vi "Main.vi"() -> ()   [LabVIEW 2015]
doc: "使用该模板构建简单状态机设计模式。各状态执行代码并决定转移状态。"
uses:
  C:/Program Files (x86)/MVS/Development/DotNet/AnyCpu/MvCamCtrl.Net.dll
  DotNet/AnyCpu/MvCamCtrl.Net.dll
  controls/RetureState.ctl
panel:
  out "FrameNum":u32 caption="图像数"
  out "ResultingFrameRate":sgl caption="采集帧率："
  out "Processed Frame":dbl caption="处理帧率："
  out "?":T1(plugin-control)
  in  "SetParam":bool
  in  "GetParam":bool caption="获取参数"
  out "error out":T2 caption="错误输出" {"code" format="%x"}
  out "CFrameoutEx":refnum<k24>
  out "PayloadSize":u32 caption="帧负载大小："
  out "CFloatValue":refnum<k24>
  out "CEnumValue":refnum<k24>
  out "CIntValue":refnum<k24>
  out "Width":u32 caption="图像宽："
  out "Height":u32 caption="图像高："
  in  "error in":errorcluster caption="错误输入" {"code" format="%x"}
  out "CCameraInfoList":refnum<k24>
  in  "PixelFormat":u32 caption="像素格式" format="%x"
  in  "Gain":sgl caption="增益(dB)" min=0 max=20 format="%.4f"
  in  "ExposureTime":sgl=5.0 caption="曝光时间(us)" min=5 max=100000 format="%.4f"
  in  "TriggerSoftWare":bool
  in  "AcquisitionStop":bool
  in  "TriggerMode":bool
  in  "Continuous":bool
  in  "AcquisitionStart":bool caption="开始采集"
  out "GrabbingStatus":bool caption="图像采集"
  out "OpenSatatus":bool caption="相机打开"
  in  "退出":bool
  in  "CloseDevice":bool
  in  "OpenDevice":bool
  in  "EumDevice":bool
  in  "DeviceList":u16(ring) caption="设备列表" items=["[GigE]MV-CA013-20GC（Vir26769280）", "[GigE]MV-CA050-10GC（Vir26769488）", "[GigE]MV-CA060-11GM（Vir26769777）", "[GigE]MV-CL020-40GM（Vir26770200）", "[GigE]MV-CL042-91GC（Vir26770020）", "[U3V]MV-CA003-21UC（Vir26771277）", "[U3V]MV-CH120-10UC（Vir26771865）", "[U3V]MV-CH120-10UM（Vir26772137）"]
  out "DeviceNum":dbl caption="设备个数"
  out "CCamera":refnum<k24>
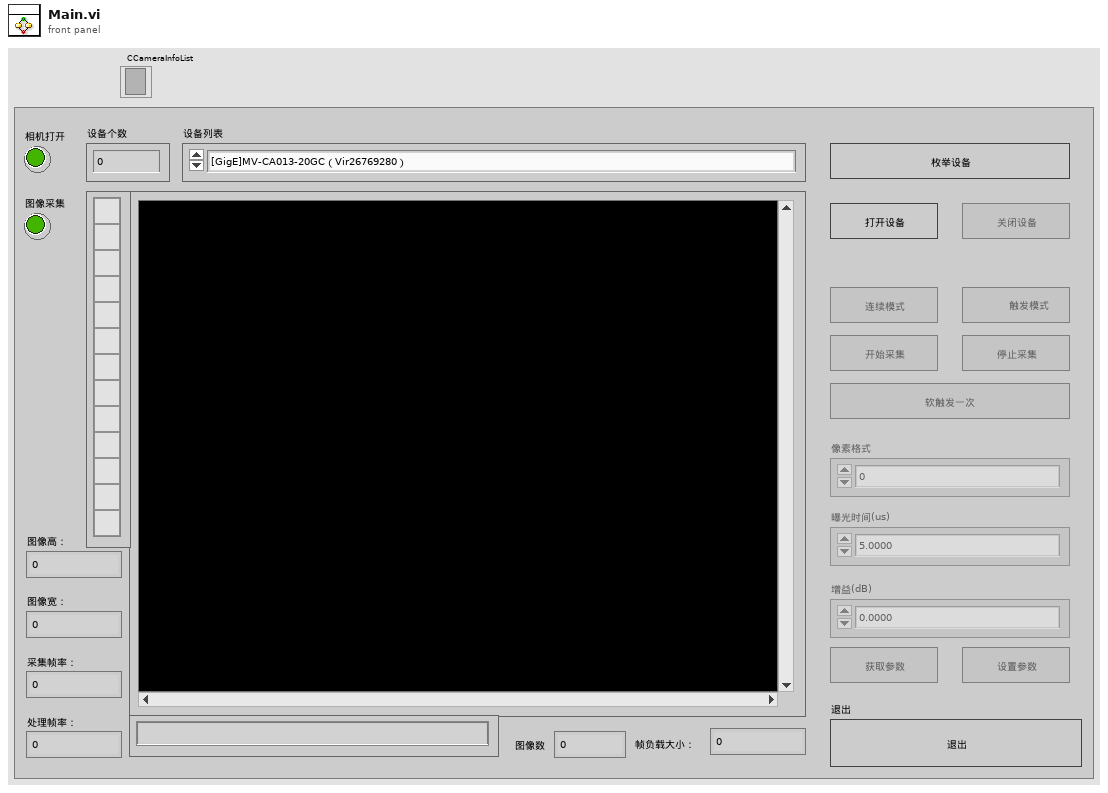
[diagram p1: front panel]
types:
  T1 = typedef "IMAQ Image.ctl" = refnum<image>
  T2 = typedef "RetureState.ctl" = errorcluster
  T3 = enum8{"Enabled", "Disabled", "Disabled and Grayed Out"}
  T4 = typedef "Image Type" = u32
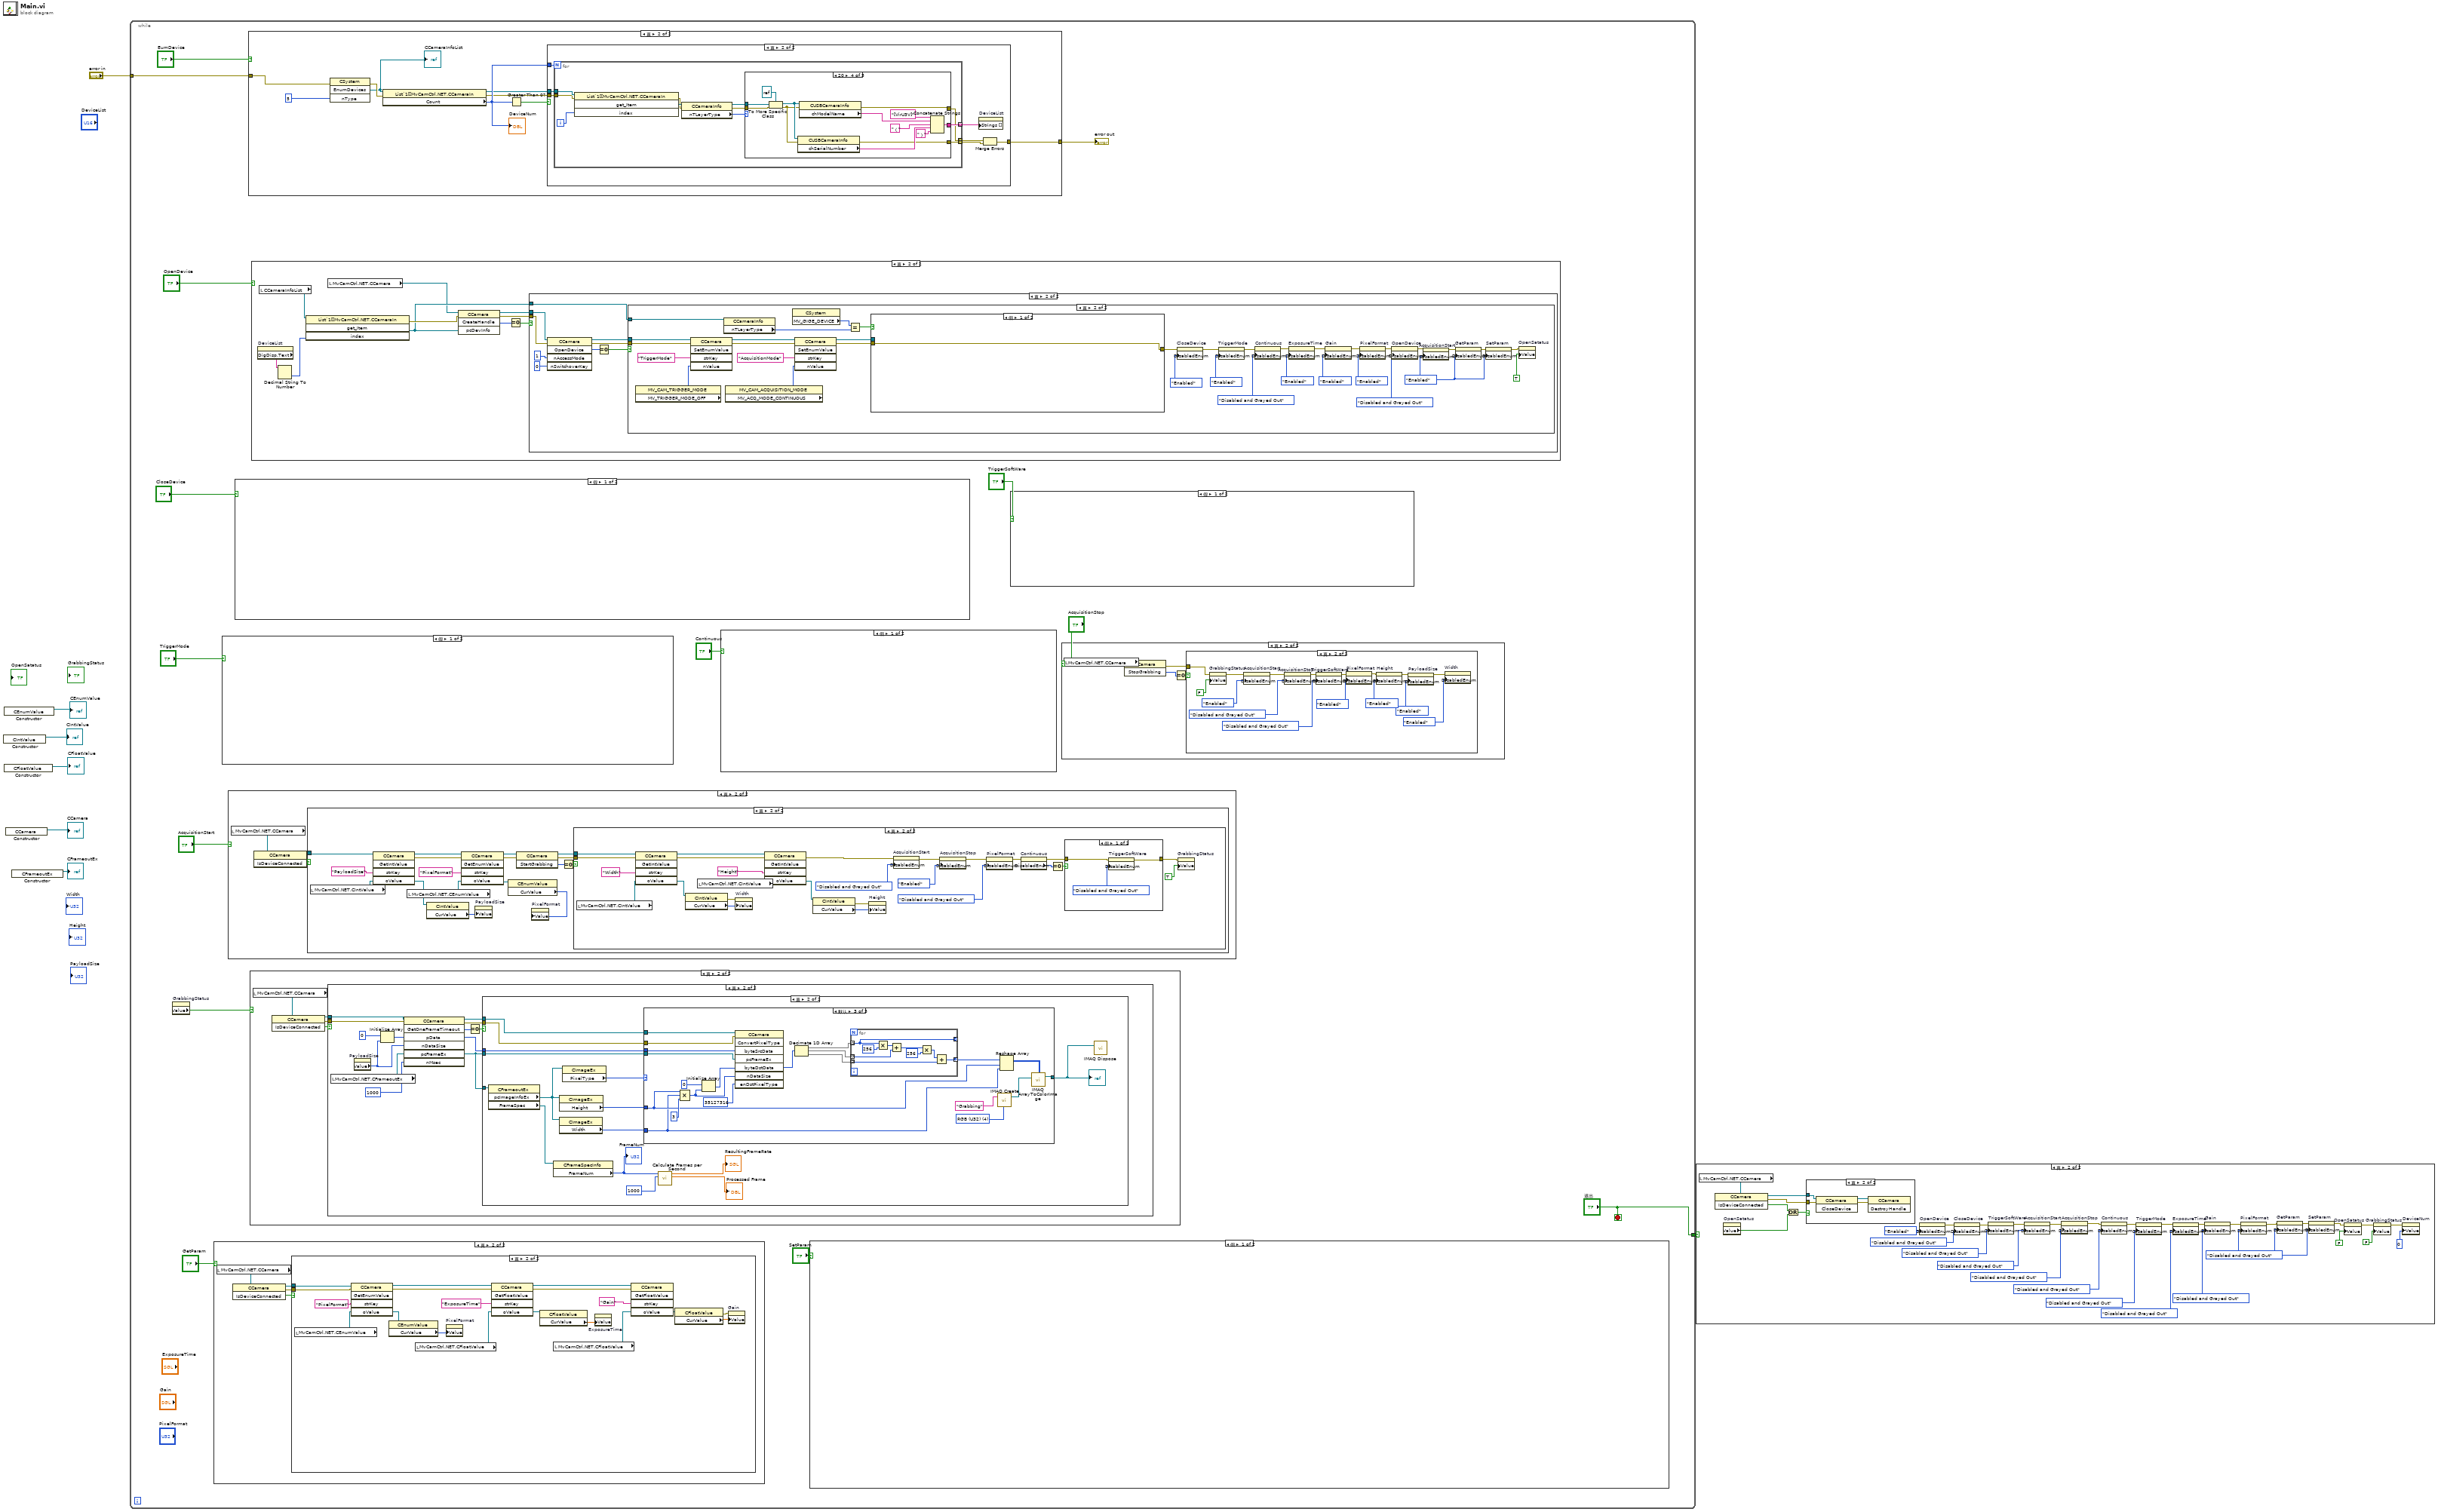
[diagram p0: block diagram]
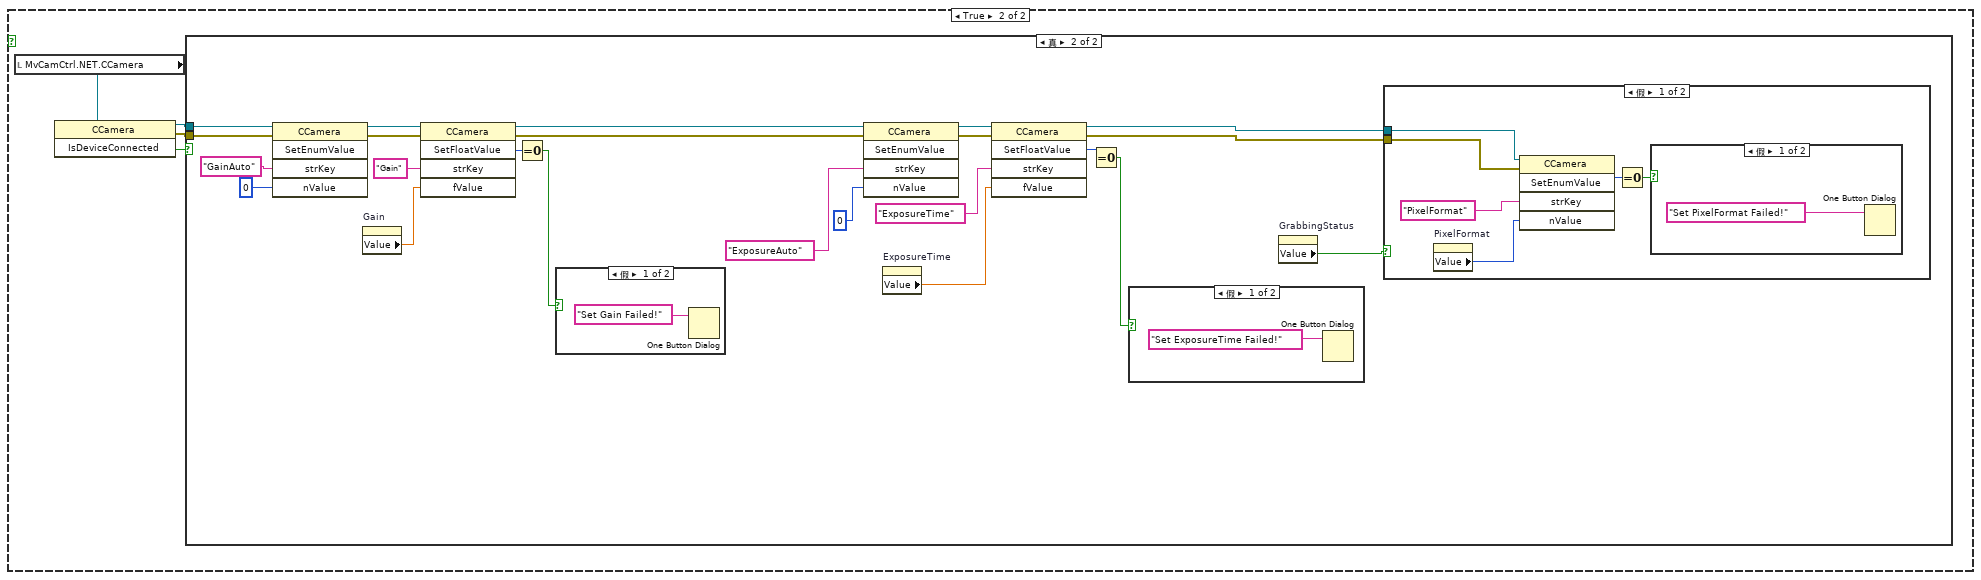
[diagram p4: hidden frame]
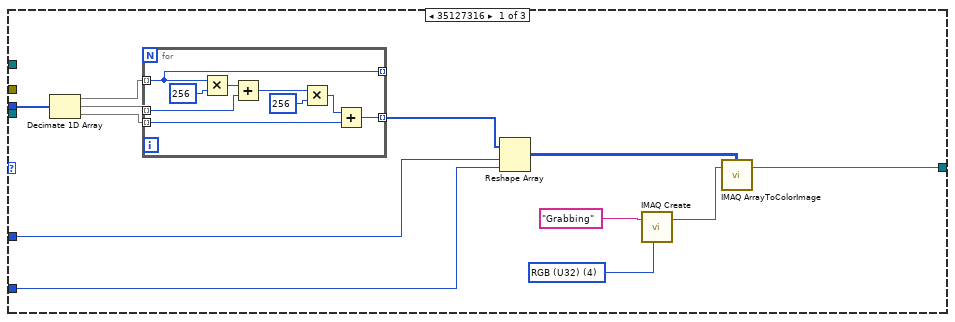
[diagram p15: hidden frame]
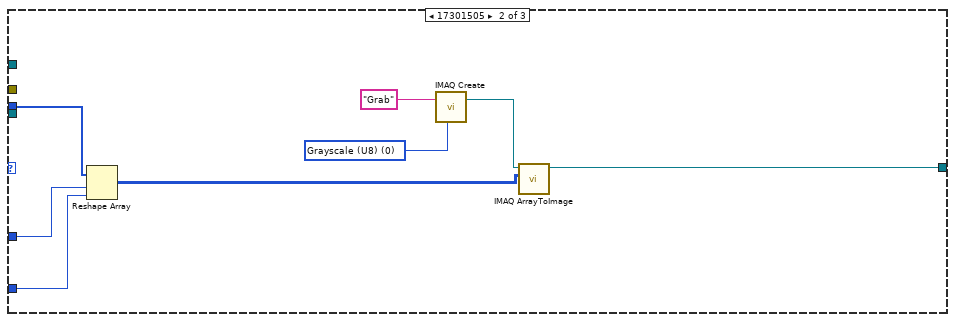
[diagram p16: hidden frame]
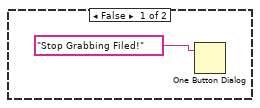
[diagram p18: hidden frame]
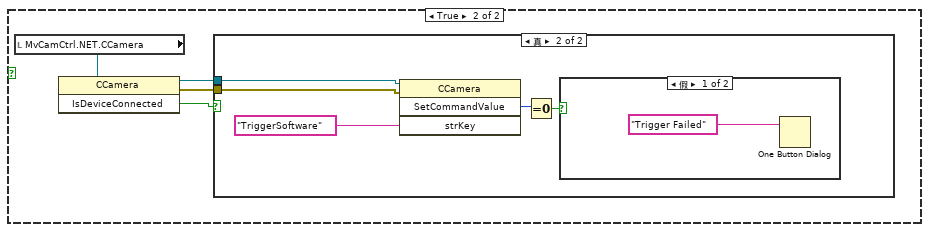
[diagram p19: hidden frame]
diagram:
  n1 = constructor class="CIntValue"() -> (reference out=→"CIntValue":refnum<k24>)  [unwired: 3 in, 2 out]
  n2 = constructor class="CEnumValue"() -> (reference out=→"CEnumValue":refnum<k24>)  [unwired: 3 in, 2 out]
  n3 = constructor class="CFloatValue"() -> (reference out=→"CFloatValue":refnum<k24>)  [unwired: 3 in, 2 out]
  n4 = constructor class="CCamera"() -> (reference out=→"CCamera":refnum<k24>)  [unwired: 3 in, 2 out]
  n5 = constructor class="CFrameoutEx"() -> (reference out=→"CFrameoutEx":refnum<k24>)  [unwired: 3 in, 2 out]
  n6 = while {
    tunnel: ["退出"] -> w7
    tunnel: "error in" -> [w13]
    stop <- "退出" stop-if-true
    n7 = property on="GrabbingStatus" class="Bool (严格)"() -> ("Value"=w12:bool)  [unwired: 2 in, 2 out]
    n8 = case shown="真" "GetParam" {
      frame False {
      }
      frame True {
        n9 = local read "CCamera"() -> (w61:refnum<k24>)
        n10 = invoke class="CCamera" method="IsDeviceConnected"(reference=w61) -> (reference out=w59:refnum<k24>, error out=w58:errorcluster, "IsDeviceConnected"=w60:bool)  [unwired: 2 in]
        n11 = case shown="真" w60 {
          tunnel: w59 -> [_ w71]
          tunnel: w58 -> [_ w70]
          frame False {
          }
          frame True {
            n12 = local read "CEnumValue"() -> (w72:refnum<k24>)
            n13 = invoke on="调用节点" class="CCamera" method="GetEnumValue"(reference=w71, error in=w70, "strKey"="PixelFormat", "oValue"=w72) -> (reference out=w78:refnum<k24>, error out=w75:errorcluster, "oValue"=w79:refnum<k24>)  [unwired: 1 in, 2 out]
            n14 = property on="属性节点" class="CEnumValue"(reference=w79) -> ("CurValue"=w80:u32)  [unwired: 1 in, 2 out]
            n15 = local read "CFloatValue"() -> (w69:refnum<k24>)
            n16 = property on="PixelFormat" class="DigNum (严格)"("Value"=w80) -> ()  [unwired: 2 in, 2 out]
            n17 = invoke on="调用节点" class="CCamera" method="GetFloatValue"(reference=w78, error in=w75, "strKey"="ExposureTime", "oValue"=w69) -> (reference out=w77:refnum<k24>, error out=w74:errorcluster, "oValue"=w63:refnum<k24>)  [unwired: 1 in, 2 out]
            n18 = property on="属性节点" class="CFloatValue"(reference=w63) -> ("CurValue"=w62:sgl)  [unwired: 1 in, 2 out]
            n19 = local read "CFloatValue"() -> (w66:refnum<k24>)
            n20 = property on="ExposureTime" class="DigNum (严格)"("Value"=w62) -> ()  [unwired: 2 in, 2 out]
            n21 = invoke on="调用节点" class="CCamera" method="GetFloatValue"(reference=w77, error in=w74, "strKey"="Gain", "oValue"=w66) -> ("oValue"=w76:refnum<k24>)  [unwired: 1 in, 4 out]
            n22 = property on="属性节点" class="CFloatValue"(reference=w76) -> (error out=w65:errorcluster, "CurValue"=w64:sgl)  [unwired: 1 in, 1 out]
            n23 = property on="Gain" class="DigNum (严格)"(error in=w65, "Value"=w64) -> ()  [unwired: 1 in, 2 out]
          }
        }
      }
    }
    n24 = case shown="假" "TriggerMode" {
      frame False {
      }
      frame True {
        n25 = local read "CCamera"() -> (w222:refnum<k24>)
        n26 = property class="MV_CAM_TRIGGER_MODE"() -> ("MV_TRIGGER_MODE_ON"=w221:i32)  [unwired: 2 in, 2 out]
        n27 = invoke class="CCamera" method="SetEnumValue"(reference=w222, "strKey"="TriggerMode", "nValue"=w221) -> (reference out=w220:refnum<k24>, error out=w219:errorcluster, "SetEnumValue"=w217:i32)  [unwired: 2 in, 2 out]
        n28 = Equal To 0?(x=w217) -> (x = 0?=w218:bool)
        n29 = case shown="真" w218 {
          tunnel: w220 -> [_ w233]
          tunnel: w219 -> [_ w232]
          frame False {
            n30 = One Button Dialog(message="Set TiggerMode Filed!") -> ()  [unwired: 1 in, 1 out]
          }
          frame True {
            n31 = property class="MV_CAM_TRIGGER_SOURCE"() -> ("MV_TRIGGER_SOURCE_SOFTWARE"=w225:i32)  [unwired: 2 in, 2 out]
            n32 = invoke class="CCamera" method="SetEnumValue"(reference=w233, error in=w232, "strKey"="TriggerSource", "nValue"=w225) -> (error out=w231:errorcluster)  [unwired: 1 in, 4 out]
            n33 = property on="Continuous" class="Bool"(error in=w231, "DisabledEnum"=T3."Enabled" ("禁用")) -> (error out=w230:errorcluster)  [unwired: 1 in, 1 out]
            n34 = property on="TriggerMode" class="Bool"(error in=w230, "DisabledEnum"=T3."Disabled and Grayed Out" ("禁用")) -> (error out=w229:errorcluster)  [unwired: 1 in, 1 out]
            n35 = property on="TriggerSoftWare" class="Bool"(error in=w229, "DisabledEnum"=T3."Enabled" ("禁用")) -> ()  [unwired: 1 in, 2 out]
          }
        }
      }
    }
    n36 = case shown="真" "AcquisitionStart" {
      frame False {
      }
      frame True {
        n37 = local read "CCamera"() -> (w236:refnum<k24>)
        n38 = invoke class="CCamera" method="IsDeviceConnected"(reference=w236) -> (reference out=w234:refnum<k24>, "IsDeviceConnected"=w235:bool)  [unwired: 2 in, 1 out]
        n39 = case shown="真" w235 {
          tunnel: w234 -> [_ w238]
          frame False {
          }
          frame True {
            n40 = local read "CIntValue"() -> (w249:refnum<k24>)
            n41 = invoke class="CCamera" method="GetIntValue"(reference=w238, "strKey"="PayloadSize", "oValue"=w249) -> (reference out=w244:refnum<k24>, error out=w242:errorcluster, "oValue"=w253:refnum<k24>)  [unwired: 2 in, 2 out]
            n42 = local read "CEnumValue"() -> (w247:refnum<k24>)
            n43 = property class="CIntValue"(reference=w253) -> ("CurValue"=w248:i64)  [unwired: 1 in, 2 out]
            n44 = invoke on="调用节点" class="CCamera" method="GetEnumValue"(reference=w244, error in=w242, "strKey"="PixelFormat", "oValue"=w247) -> (reference out=w243:refnum<k24>, error out=w241:errorcluster, "oValue"=w246:refnum<k24>)  [unwired: 1 in, 2 out]
            n45 = property on="PayloadSize" class="DigNum (严格)"("Value"=w248) -> ()  [unwired: 2 in, 2 out]
            n46 = property class="CEnumValue"(reference=w246) -> ("CurValue"=w245:u32)  [unwired: 1 in, 2 out]
            n47 = invoke class="CCamera" method="StartGrabbing"(reference=w243, error in=w241) -> (reference out=w251:refnum<k24>, error out=w250:errorcluster, "StartGrabbing"=w237:i32)  [unwired: 1 in]
            n48 = property on="PixelFormat" class="DigNum (严格)"("Value"=w245) -> ()  [unwired: 2 in, 2 out]
            n49 = Equal To 0?(x=w237) -> (x = 0?=w252:bool)
            n50 = case shown="真" w252 {
              tunnel: w251 -> [_ w280]
              tunnel: w250 -> [_ w277]
              frame False {
                n51 = One Button Dialog(message="Satrt Grabbing Failed") -> ()  [unwired: 1 in, 1 out]
              }
              frame True {
                n52 = local read "CIntValue"() -> (w258:refnum<k24>)
                n53 = invoke class="CCamera" method="GetIntValue"(reference=w280, error in=w277, "strKey"="Width", "oValue"=w258) -> (reference out=w279:refnum<k24>, error out=w278:errorcluster, "oValue"=w275:refnum<k24>)  [unwired: 1 in, 2 out]
                n54 = property class="CIntValue"(reference=w275) -> (error out=w276:errorcluster, "CurValue"=w274:i64)  [unwired: 1 in, 1 out]
                n55 = local read "CIntValue"() -> (w257:refnum<k24>)
                n56 = property on="Width" class="DigNum (严格)"(error in=w276, "Value"=w274) -> ()  [unwired: 1 in, 2 out]
                n57 = invoke class="CCamera" method="GetIntValue"(reference=w279, error in=w278, "strKey"="Height", "oValue"=w257) -> (error out=w260:errorcluster, "oValue"=w264:refnum<k24>)  [unwired: 1 in, 3 out]
                n58 = property class="CIntValue"(reference=w264) -> (error out=w273:errorcluster, "CurValue"=w272:i64)  [unwired: 1 in, 1 out]
                n59 = property on="Height" class="DigNum (严格)"(error in=w273, "Value"=w272) -> ()  [unwired: 1 in, 2 out]
                n60 = property on="AcquisitionStart" class="Bool"(error in=w260, "DisabledEnum"=T3."Disabled and Grayed Out" ("禁用")) -> (error out=w271:errorcluster)  [unwired: 1 in, 1 out]
                n61 = property on="AcquisitionStop" class="Bool"(error in=w271, "DisabledEnum"=T3."Enabled" ("禁用")) -> (error out=w263:errorcluster)  [unwired: 1 in, 1 out]
                n62 = property on="PixelFormat" class="DigNum (严格)"(error in=w263, "DisabledEnum"=T3."Disabled and Grayed Out" ("禁用")) -> (error out=w259:errorcluster)  [unwired: 1 in, 1 out]
                n63 = property on="Continuous" class="Bool"(error in=w259) -> (error out=w270:errorcluster, "DisabledEnum"=w265:T3)  [unwired: 1 in, 1 out]
                n64 = Equal To 0?(x=w265) -> (x = 0?=w266:bool)
                n65 = case shown="假" w266 {
                  tunnel: w270 -> [w282 w286]
                  tunnel: [w281 w285] -> w268
                  frame False {
                    n66 = property on="TriggerSoftWare" class="Bool"(error in=w282, "DisabledEnum"=T3."Disabled and Grayed Out" ("禁用")) -> (error out=w281:errorcluster)  [unwired: 1 in, 1 out]
                  }
                  frame True {
                    n67 = property on="TriggerSoftWare" class="Bool"(error in=w286, "DisabledEnum"=T3."Enabled" ("禁用")) -> (error out=w285:errorcluster)  [unwired: 1 in, 1 out]
                  }
                }
                n68 = property on="GrabbingStatus" class="Bool (严格)"(error in=w268, "Value"=TRUE) -> ()  [unwired: 1 in, 2 out]
              }
            }
          }
        }
      }
    }
    n69 = case shown="假" "CloseDevice" {
      frame False {
      }
      frame True {
        n70 = local read "CCamera"() -> (w448:refnum<k24>)
        n71 = invoke class="CCamera" method="IsDeviceConnected"(reference=w448) -> (reference out=w447:refnum<k24>, error out=w446:errorcluster, "IsDeviceConnected"=w445:bool)  [unwired: 2 in]
        n72 = case shown="真" w445 {
          tunnel: w447 -> [_ w454]
          tunnel: w446 -> [_ w453]
          frame False {
          }
          frame True {
            w452 = T3."Disabled and Grayed Out" ("禁用")
            n73 = invoke class="CCamera" method="CloseDevice"(reference=w454, error in=w453) -> (reference out=w478:refnum<k24>, error out=w477:errorcluster)  [unwired: 1 in, 1 out]
            n74 = invoke class="CCamera" method="DestroyHandle"(reference=w478, error in=w477) -> (error out=w476:errorcluster)  [unwired: 1 in, 2 out]
            n75 = property on="OpenDevice" class="Bool"(error in=w476, "DisabledEnum"=T3."Enabled" ("禁用")) -> (error out=w472:errorcluster)  [unwired: 1 in, 1 out]
            n76 = property on="CloseDevice" class="Bool"(error in=w472, "DisabledEnum"=T3."Disabled and Grayed Out" ("禁用")) -> (error out=w471:errorcluster)  [unwired: 1 in, 1 out]
            n77 = property on="Continuous" class="Bool"(error in=w471, "DisabledEnum"=T3."Disabled and Grayed Out" ("禁用")) -> (error out=w470:errorcluster)  [unwired: 1 in, 1 out]
            n78 = property on="TriggerMode" class="Bool"(error in=w470, "DisabledEnum"=T3."Disabled and Grayed Out" ("禁用")) -> (error out=w457:errorcluster)  [unwired: 1 in, 1 out]
            n79 = property on="AcquisitionStop" class="Bool"(error in=w457, "DisabledEnum"=T3."Disabled and Grayed Out" ("禁用")) -> (error out=w469:errorcluster)  [unwired: 1 in, 1 out]
            n80 = property on="AcquisitionStart" class="Bool"(error in=w469, "DisabledEnum"=T3."Disabled and Grayed Out" ("禁用")) -> (error out=w455:errorcluster)  [unwired: 1 in, 1 out]
            n81 = property on="TriggerSoftWare" class="Bool"(error in=w455, "DisabledEnum"=T3."Disabled and Grayed Out" ("禁用")) -> (error out=w459:errorcluster)  [unwired: 1 in, 1 out]
            n82 = property on="PixelFormat" class="DigNum (严格)"(error in=w459, "DisabledEnum"=T3."Disabled and Grayed Out" ("禁用")) -> (error out=w458:errorcluster)  [unwired: 1 in, 1 out]
            n83 = property on="Gain" class="DigNum (严格)"(error in=w458, "DisabledEnum"=T3."Disabled and Grayed Out" ("禁用")) -> (error out=w468:errorcluster)  [unwired: 1 in, 1 out]
            n84 = property on="ExposureTime" class="DigNum (严格)"(error in=w468, "DisabledEnum"=w452) -> (error out=w451:errorcluster)  [unwired: 1 in, 1 out]
            n85 = property on="GetParam" class="Bool"(error in=w451, "DisabledEnum"=w452) -> (error out=w450:errorcluster)  [unwired: 1 in, 1 out]
            n86 = property on="SetParam" class="Bool"(error in=w450, "DisabledEnum"=w452) -> (error out=w449:errorcluster)  [unwired: 1 in, 1 out]
            n87 = property on="OpenSatatus" class="Bool (严格)"(error in=w449, "Value"=FALSE) -> (error out=w460:errorcluster)  [unwired: 1 in, 1 out]
            n88 = property on="GrabbingStatus" class="Bool (严格)"(error in=w460, "Value"=FALSE) -> ()  [unwired: 1 in, 2 out]
          }
        }
      }
    }
    n89 = case shown="真" "EumDevice" {
      tunnel: w13 -> [w360 w367]
      tunnel: [w360 w364] -> w11
      frame False {
      }
      frame True {
        n90 = invoke on="调用节点" class="CSystem" method="EnumDevices"(error in=w367, "nType"=u32 5) -> (error out=w366:errorcluster, "EnumDevices"=w361:refnum<k24>)  [unwired: 2 in, 2 out]
        "CCameraInfoList" <- w361
        n91 = property on="属性节点" class="List`1[[MvCamCtrl.NET.CCameraIn"(reference=w361, error in=w366) -> (reference out=w363:refnum<k24>, error out=w365:errorcluster, "Count"=w368:i32)
        "DeviceNum" <- w368
        n92 = Greater Than 0?(x=w368) -> (x > 0?=w369:bool)
        n93 = case shown="真" w369 {
          tunnel: w368 -> [_ w379]
          tunnel: w363 -> [_ w378]
          tunnel: w365 -> [w370 w376]
          tunnel: [w370 w373] -> w364
          frame False {
            n94 = One Button Dialog(message="Not Found Devices!", button name ("OK")="Warning") -> ()  [unwired: 1 out]
          }
          frame True {
            n95 = for {
              N: w379 -> [_]
              tunnel: [w390] -> w377 mode=indexing
              tunnel: w378 -> [w385]
              tunnel: w376 -> [w384]
              tunnel: [w381] -> w375 mode=indexing
              tunnel: [w380] -> w374 mode=indexing
              i -> [w389]
              n96 = invoke class="List`1[[MvCamCtrl.NET.CCameraIn" method="get_Item"(reference=w385, error in=w384, "index"=w389) -> (error out=w383:errorcluster, "get_Item"=w386:refnum<k24>)  [unwired: 1 in, 2 out]
              n97 = property class="CCameraInfo"(reference=w386, error in=w383) -> (reference out=w387:refnum<k24>, error out=w382:errorcluster, "nTLayerType"=w388:u32)
              n98 = case shown="20" w388 {
                tunnel: ["UnsupportDev" w402 w406 w419 w439] -> w390
                tunnel: w387 -> [_ w398 w410 w423 w437]
                tunnel: w382 -> [w391 w396 w409 w422 w433]
                tunnel: [w391 w394 w407 w421 w435] -> w381
                tunnel: [w391 w393 w408 w420 w434] -> w380
                frame 0, Default {
                }
                frame 1 {
                  n99 = To More Specific Class(target class=refnum<k24> refnum ("CGigECameraInfo"), reference=w398, error in=w396) -> (specific class reference=w397:refnum<k24>, error out=w395:errorcluster)
                  n100 = property class="CGigECameraInfo"(reference=w397, error in=w395) -> (error out=w394:errorcluster, "chModelName"=w401:string)  [unwired: 1 out]
                  n101 = property class="CGigECameraInfo"(reference=w397, error in=w395) -> (error out=w393:errorcluster, "chSerialNumber"=w403:string)  [unwired: 1 out]
                  n102 = Concatenate Strings("[GigE]" ("字符串"), w401, "（" ("字符串"), w403, "）" ("字符串")) -> (w402:string)
                }
                frame 16 {
                  n103 = To More Specific Class(target class=refnum<k24> refnum ("CGigECameraInfo"), reference=w410, error in=w409) -> (specific class reference=w412:refnum<k24>, error out=w411:errorcluster)
                  n104 = property class="CGigECameraInfo"(reference=w412, error in=w411) -> (error out=w407:errorcluster, "chModelName"=w415:string)  [unwired: 1 out]
                  n105 = property class="CGigECameraInfo"(reference=w412, error in=w411) -> (error out=w408:errorcluster, "chSerialNumber"=w416:string)  [unwired: 1 out]
                  n106 = Concatenate Strings("[VirGigE]" ("字符串"), w415, "（" ("字符串"), w416, "）" ("字符串")) -> (w406:string)
                }
                frame 32 {
                  n107 = To More Specific Class(target class=refnum<k24> refnum ("CUSBCameraInfo"), reference=w423, error in=w422) -> (specific class reference=w425:refnum<k24>, error out=w424:errorcluster)
                  n108 = property class="CUSBCameraInfo"(reference=w425, error in=w424) -> (error out=w420:errorcluster, "chSerialNumber"=w429:string)  [unwired: 1 out]
                  n109 = property class="CUSBCameraInfo"(reference=w425, error in=w424) -> (error out=w421:errorcluster, "chModelName"=w428:string)  [unwired: 1 out]
                  n110 = Concatenate Strings("[VirU3V]" ("字符串"), w428, "（" ("字符串"), w429, "）" ("字符串")) -> (w419:string)
                }
                frame 4 {
                  n111 = To More Specific Class(target class=refnum<k24> refnum ("CUSBCameraInfo"), reference=w437, error in=w433) -> (specific class reference=w436:refnum<k24>, error out=w432:errorcluster)
                  n112 = property class="CUSBCameraInfo"(reference=w436, error in=w432) -> (error out=w434:errorcluster, "chSerialNumber"=w442:string)  [unwired: 1 out]
                  n113 = property class="CUSBCameraInfo"(reference=w436, error in=w432) -> (error out=w435:errorcluster, "chModelName"=w441:string)  [unwired: 1 out]
                  n114 = Concatenate Strings("[U3V]" ("字符串"), w441, "（" ("字符串"), w442, "）" ("字符串")) -> (w439:string)
                }
              }
            }
            n115 = property on="DeviceList" class="Ring (严格)"("Strings []"=w377) -> ()  [unwired: 2 in, 2 out]
            n116 = Merge Errors(w375, w374) -> (w373:errorcluster)
          }
        }
      }
    }
    "error out" <- w11
    n117 = case shown="真" w12 {
      frame False {
      }
      frame True {
        n118 = local read "CCamera"() -> (w84:refnum<k24>)
        n119 = invoke class="CCamera" method="IsDeviceConnected"(reference=w84) -> (reference out=w82:refnum<k24>, error out=w81:errorcluster, "IsDeviceConnected"=w83:bool)  [unwired: 2 in]
        n120 = case shown="真" w83 {
          tunnel: w82 -> [_ w89]
          tunnel: w81 -> [_ w88]
          frame False {
          }
          frame True {
            n121 = local read "CFrameoutEx"() -> (w95:refnum<k24>)
            n122 = property on="PayloadSize" class="DigNum (严格)"() -> ("Value"=w91:u32)  [unwired: 2 in, 2 out]
            n123 = Initialize Array(0, w91) -> (w93:i32[])
            n124 = invoke class="CCamera" method="GetOneFrameTimeout"(reference=w89, error in=w88, "pData"=w93, "nDataSize"=w91, "pcFrameEx"=w95, "nMsec"=1000) -> (reference out=w87:refnum<k24>, error out=w94:errorcluster, "GetOneFrameTimeout"=w97:i32, "pData"=w90:u8[], "pcFrameEx"=w86:refnum<k24>)  [unwired: 1 in, 2 out]
            n125 = Equal To 0?(x=w97) -> (x = 0?=w96:bool)
            n126 = case shown="真" w96 {
              tunnel: w86 -> [_ w111]
              tunnel: w94 -> [_ w112]
              tunnel: w90 -> [_ w105]
              tunnel: w87 -> [_ w103]
              tunnel: w86 -> [_ w102]
              frame False {
              }
              frame True {
                n127 = property on="属性节点" class="CFrameoutEx"(reference=w111) -> ("pcImageInfoEx"=w107:refnum<k24>, "FrameSpec"=w104:refnum<k24>)  [unwired: 1 in, 2 out]
                n128 = property on="属性节点" class="CFrameSpecInfo"(reference=w104) -> ("FrameNum"=w101:u32)  [unwired: 1 in, 2 out]
                "FrameNum" <- w101
                n129 = property on="属性节点" class="CImageEx"(reference=w107) -> ("Width"=w110:u16)  [unwired: 1 in, 2 out]
                n130 = property on="属性节点" class="CImageEx"(reference=w107) -> ("Height"=w109:u16)  [unwired: 1 in, 2 out]
                n131 = property on="属性节点" class="CImageEx"(reference=w107) -> ("PixelType"=w108:i32)  [unwired: 1 in, 2 out]
                n132 = case shown="默认" w108 {
                  tunnel: w105 -> [w120 w141 w155]
                  tunnel: w109 -> [w115 w140 w143]
                  tunnel: w110 -> [w114 w139 w142]
                  tunnel: w112 -> [_ _ w152]
                  tunnel: [w124 w134 w161] -> w106
                  tunnel: w103 -> [_ _ w156]
                  tunnel: w102 -> [_ _ w145]
                  frame 35127316 {
                    w122 = T4 4 items=["Grayscale (U8)", "Grayscale (I16)", "Grayscale (SGL)", "Complex (CSG)", "RGB (U32)", "HSL (U32)", "RGB (U64)", "Grayscale (U16)"] ("Image Type")
                    n133 = Decimate 1D Array(w120) -> (w119:u8[], w118:u8[], w117:u8[])
                    n134 = for {
                      tunnel: [w125] -> _ mode=indexing
                      tunnel: w118 -> [w128] mode=indexing
                      tunnel: w117 -> [w127] mode=indexing
                      tunnel: [w126] -> w116 mode=indexing
                      tunnel: w119 -> [w125] mode=indexing
                      n135 = Multiply(x=w125, y=u16 256) -> (x*y=w132:u16)
                      n136 = Add(x=w132, y=w128) -> (x+y=w129:u16)
                      n137 = Multiply ("乘")(x=w129, y=u16 256) -> (x*y=w131:u32)
                      n138 = Add(x=w131, y=w127) -> (x+y=w126:u32)
                    }
                    n139 = Reshape Array(w116, w115, w114) -> (w113:u32[][])
                    n140 = call "IMAQ Create"("Image Name"="Grabbing", "Image Type"=w122) -> ("New Image"=w121:T1)  [unwired: 3 in, 1 out]
                    n141 = call "IMAQ ArrayToColorImage"("Image Pixels (U32)"=w113, "Image"=w121) -> ("Image Out"=w124:T1)  [unwired: 3 in, 1 out]
                  }
                  frame 17301505 {
                    w137 = T4 0 items=["Grayscale (U8)", "Grayscale (I16)", "Grayscale (SGL)", "Complex (CSG)", "RGB (U32)", "HSL (U32)", "RGB (U64)", "Grayscale (U16)"] ("Image Type")
                    n142 = Reshape Array(w141, w140, w139) -> (w135:u8[][])
                    n143 = call "IMAQ Create"("Image Name"="Grab", "Image Type"=w137) -> ("New Image"=w136:T1)  [unwired: 3 in, 1 out]
                    n144 = call "IMAQ ArrayToImage"("Image Pixels (U8)"=w135, "Image"=w136) -> ("Image Out"=w134:T1)  [unwired: 8 in, 1 out]
                  }
                  frame Default {
                    w159 = T4 4 items=["Grayscale (U8)", "Grayscale (I16)", "Grayscale (SGL)", "Complex (CSG)", "RGB (U32)", "HSL (U32)", "RGB (U64)", "Grayscale (U16)"] ("Image Type")
                    n145 = Compound Arithmetic op=MULTIPLY(w143, w142, 3) -> (w153:i32)
                    n146 = Initialize Array(0, w153) -> (w154:i32[])
                    n147 = invoke class="CCamera" method="ConvertPixelType"(reference=w156, error in=w152, "byteSrcData"=w155, "pcFrameEx"=w145, "byteDstData"=w154, "nDataSize"=w153, "enDstPixelType"=u32 35127316) -> ("byteDstData"=w144:u8[])  [unwired: 1 in, 7 out]
                    n148 = Decimate 1D Array(w144) -> (w149:u8[], w148:u8[], w147:u8[])
                    n149 = for {
                      tunnel: [w163] -> _ mode=indexing
                      tunnel: w148 -> [w166] mode=indexing
                      tunnel: w147 -> [w165] mode=indexing
                      tunnel: [w164] -> w157 mode=indexing
                      tunnel: w149 -> [w163] mode=indexing
                      n150 = Multiply(x=w163, y=u16 256) -> (x*y=w170:u16)
                      n151 = Add(x=w170, y=w166) -> (x+y=w167:u16)
                      n152 = Multiply ("乘")(x=w167, y=u16 256) -> (x*y=w169:u32)
                      n153 = Add(x=w169, y=w165) -> (x+y=w164:u32)
                    }
                    n154 = call "IMAQ Create"("Image Name"="Grabbing", "Image Type"=w159) -> ("New Image"=w162:T1)  [unwired: 3 in, 1 out]
                    n155 = Reshape Array(w157, w143, w142) -> (w158:u32[][])
                    n156 = call "IMAQ ArrayToColorImage"("Image Pixels (U32)"=w158, "Image"=w162) -> ("Image Out"=w161:T1)  [unwired: 3 in, 1 out]
                  }
                }
                "?" <- w106
                n157 = call <vilib>:"Calculate Frames per Second.vi"("Update Interval (ms)"=1000, "Buffer Number"=w101) -> ("Processed Frames/s"=→"Processed Frame":dbl, "Acquired Frames/s"=→"ResultingFrameRate":dbl)  [unwired: 7 in, 1 out]
                n158 = call "IMAQ Dispose"("Image"=w106) -> ()  [unwired: 5 in, 1 out]
              }
            }
          }
        }
      }
    }
    n159 = case shown="真" "OpenDevice" {
      frame False {
      }
      frame True {
        n160 = property on="DeviceList" class="Ring (严格)"() -> ("DigDisp.Text"=w296:string)  [unwired: 2 in, 2 out]
        n161 = local read "CCameraInfoList"() -> (w287:refnum<k24>)
        n162 = Decimal String To Number(string=w296) -> (number=w295:i32)  [unwired: 2 in, 1 out]
        n163 = invoke class="List`1[[MvCamCtrl.NET.CCameraIn" method="get_Item"(reference=w287, "index"=w295) -> (error out=w294:errorcluster, "get_Item"=w293:refnum<k24>)  [unwired: 2 in, 2 out]
        n164 = local read "CCamera"() -> (w291:refnum<k24>)
        n165 = invoke class="CCamera" method="CreateHandle"(reference=w291, error in=w294, "pcDevInfo"=w293) -> (reference out=w292:refnum<k24>, error out=w290:errorcluster, "CreateHandle"=w289:i32)  [unwired: 1 in, 1 out]
        n166 = Equal To 0?(x=w289) -> (x = 0?=w288:bool)
        n167 = case shown="真" w288 {
          tunnel: w290 -> [_ w301]
          tunnel: w293 -> [_ w300]
          tunnel: w292 -> [_ w299]
          frame False {
            n168 = One Button Dialog(message="Create Camera Handle Failed!") -> ()  [unwired: 1 in, 1 out]
          }
          frame True {
            n169 = invoke class="CCamera" method="OpenDevice"(reference=w299, error in=w301, "nAccessMode"=1, "nSwitchoverKey"=0) -> (reference out=w303:refnum<k24>, error out=w302:errorcluster, "OpenDevice"=w298:i32)  [unwired: 1 in, 2 out]
            n170 = Equal To 0?(x=w298) -> (x = 0?=w306:bool)
            n171 = case shown="真" w306 {
              tunnel: w303 -> [w311 w345]
              tunnel: w302 -> [w310 w344]
              tunnel: w300 -> [_ w321]
              frame False {
                n172 = invoke class="CCamera" method="DestroyHandle"(reference=w311, error in=w310) -> (error out=w307:errorcluster)  [unwired: 1 in, 2 out]
                n173 = One Button Dialog(message="Open Failed") -> ()  [unwired: 1 in, 1 out]
                n174 = property on="OpenSatatus" class="Bool (严格)"(error in=w307, "Value"=FALSE) -> ()  [unwired: 1 in, 2 out]
              }
              frame True {
                w312 = T3."Enabled" ("禁用")
                n175 = property class="MV_CAM_TRIGGER_MODE"() -> ("MV_TRIGGER_MODE_OFF"=w338:i32)  [unwired: 2 in, 2 out]
                n176 = invoke class="CCamera" method="SetEnumValue"(reference=w345, error in=w344, "strKey"="TriggerMode", "nValue"=w338) -> (reference out=w340:refnum<k24>, error out=w339:errorcluster)  [unwired: 1 in, 3 out]
                n177 = property on="属性节点" class="CCameraInfo"(reference=w321) -> ("nTLayerType"=w343:u32)  [unwired: 1 in, 2 out]
                n178 = property class="MV_CAM_ACQUISITION_MODE"() -> ("MV_ACQ_MODE_CONTINUOUS"=w336:i32)  [unwired: 2 in, 2 out]
                n179 = property class="CSystem"() -> ("MV_GIGE_DEVICE"=w335:i32)  [unwired: 2 in, 2 out]
                n180 = invoke class="CCamera" method="SetEnumValue"(reference=w340, error in=w339, "strKey"="AcquisitionMode", "nValue"=w336) -> (reference out=w317:refnum<k24>, error out=w318:errorcluster)  [unwired: 1 in, 3 out]
                n181 = Equal?(x=w335, y=w343) -> (x = y?=w342:bool)
                n182 = case shown="假" w342 {
                  tunnel: w317 -> [_ w353]
                  tunnel: w318 -> [w346 w352]
                  tunnel: [w346 w347] -> w334
                  frame False {
                  }
                  frame True {
                    n183 = invoke class="CCamera" method="GIGE_GetOptimalPacketSize"(reference=w353, error in=w352) -> (reference out=w350:refnum<k24>, error out=w349:errorcluster, "GIGE_GetOptimalPacketSize"=w348:i32)  [unwired: 1 in]
                    n184 = Greater Than 0?(x=w348) -> (x > 0?=w351:bool)
                    n185 = case shown="假" w351 {
                      tunnel: w350 -> [_ w359]
                      tunnel: w349 -> [w354 w358]
                      tunnel: w348 -> [_ w356]
                      tunnel: [w354 w355] -> w347
                      frame False {
                      }
                      frame True {
                        n186 = invoke class="CCamera" method="SetIntValue"(reference=w359, error in=w358, "strKey"="GevSCPSPacketSize", "nValue"=w356) -> (error out=w355:errorcluster)  [unwired: 1 in, 4 out]
                      }
                    }
                  }
                }
                n187 = property on="CloseDevice" class="Bool"(error in=w334, "DisabledEnum"=T3."Enabled" ("禁用")) -> (error out=w330:errorcluster)  [unwired: 1 in, 1 out]
                n188 = property on="TriggerMode" class="Bool"(error in=w330, "DisabledEnum"=T3."Enabled" ("禁用")) -> (error out=w333:errorcluster)  [unwired: 1 in, 1 out]
                n189 = property on="Continuous" class="Bool"(error in=w333, "DisabledEnum"=T3."Disabled and Grayed Out" ("禁用")) -> (error out=w319:errorcluster)  [unwired: 1 in, 1 out]
                n190 = property on="ExposureTime" class="DigNum (严格)"(error in=w319, "DisabledEnum"=T3."Enabled" ("禁用")) -> (error out=w332:errorcluster)  [unwired: 1 in, 1 out]
                n191 = property on="Gain" class="DigNum (严格)"(error in=w332, "DisabledEnum"=T3."Enabled" ("禁用")) -> (error out=w331:errorcluster)  [unwired: 1 in, 1 out]
                n192 = property on="PixelFormat" class="DigNum (严格)"(error in=w331, "DisabledEnum"=T3."Enabled" ("禁用")) -> (error out=w323:errorcluster)  [unwired: 1 in, 1 out]
                n193 = property on="OpenDevice" class="Bool"(error in=w323, "DisabledEnum"=T3."Disabled and Grayed Out" ("禁用")) -> (error out=w320:errorcluster)  [unwired: 1 in, 1 out]
                n194 = property on="AcquisitionStart" class="Bool"(error in=w320, "DisabledEnum"=w312) -> (error out=w316:errorcluster)  [unwired: 1 in, 1 out]
                n195 = property on="GetParam" class="Bool"(error in=w316, "DisabledEnum"=w312) -> (error out=w315:errorcluster)  [unwired: 1 in, 1 out]
                n196 = property on="SetParam" class="Bool"(error in=w315, "DisabledEnum"=w312) -> (error out=w314:errorcluster)  [unwired: 1 in, 1 out]
                n197 = property on="OpenSatatus" class="Bool (严格)"(error in=w314, "Value"=TRUE ("布尔")) -> ()  [unwired: 1 in, 2 out]
              }
            }
          }
        }
      }
    }
    n198 = case shown="假" "Continuous" {
      frame False {
      }
      frame True {
        n199 = local read "CCamera"() -> (w209:refnum<k24>)
        n200 = property class="MV_CAM_TRIGGER_MODE"() -> ("MV_TRIGGER_MODE_OFF"=w208:i32)  [unwired: 2 in, 2 out]
        n201 = invoke class="CCamera" method="SetEnumValue"(reference=w209, "strKey"="TriggerMode", "nValue"=w208) -> (error out=w207:errorcluster, "SetEnumValue"=w206:i32)  [unwired: 2 in, 3 out]
        n202 = Equal To 0?(x=w206) -> (x = 0?=w205:bool)
        n203 = case shown="真" w205 {
          tunnel: w207 -> [_ w211]
          frame False {
          }
          frame True {
            n204 = property on="TriggerMode" class="Bool"(error in=w211, "DisabledEnum"=T3."Enabled" ("禁用")) -> (error out=w215:errorcluster)  [unwired: 1 in, 1 out]
            n205 = property on="Continuous" class="Bool"(error in=w215, "DisabledEnum"=T3."Disabled and Grayed Out" ("禁用")) -> (error out=w214:errorcluster)  [unwired: 1 in, 1 out]
            n206 = property on="TriggerSoftWare" class="Bool"(error in=w214, "DisabledEnum"=T3."Disabled and Grayed Out" ("禁用")) -> ()  [unwired: 1 in, 2 out]
          }
        }
      }
    }
    n207 = case shown="假" "SetParam" {
      frame False {
      }
      frame True {
        n208 = local read "CCamera"() -> (w25:refnum<k24>)
        n209 = invoke class="CCamera" method="IsDeviceConnected"(reference=w25) -> (reference out=w23:refnum<k24>, error out=w22:errorcluster, "IsDeviceConnected"=w24:bool)  [unwired: 2 in]
        n210 = case shown="真" w24 {
          tunnel: w23 -> [_ w40]
          tunnel: w22 -> [_ w39]
          frame False {
          }
          frame True {
            n211 = invoke on="调用节点" class="CCamera" method="SetEnumValue"(reference=w40, error in=w39, "strKey"="GainAuto", "nValue"=0) -> (reference out=w45:refnum<k24>, error out=w44:errorcluster)  [unwired: 1 in, 3 out]
            n212 = property on="Gain" class="DigNum (严格)"() -> ("Value"=w41:sgl)  [unwired: 2 in, 2 out]
            n213 = invoke on="调用节点" class="CCamera" method="SetFloatValue"(reference=w45, error in=w44, "strKey"="Gain", "fValue"=w41) -> (reference out=w30:refnum<k24>, error out=w27:errorcluster, "SetFloatValue"=w43:i32)  [unwired: 1 in, 2 out]
            n214 = Equal To 0?(x=w43) -> (x = 0?=w42:bool)
            n215 = case shown="假" w42 {
              frame False {
                n216 = One Button Dialog(message="Set Gain Failed!") -> ()  [unwired: 1 in, 1 out]
              }
              frame True {
              }
            }
            n217 = invoke on="调用节点" class="CCamera" method="SetEnumValue"(reference=w30, error in=w27, "strKey"="ExposureAuto", "nValue"=0) -> (reference out=w35:refnum<k24>, error out=w34:errorcluster)  [unwired: 1 in, 3 out]
            n218 = property on="ExposureTime" class="DigNum (严格)"() -> ("Value"=w26:sgl)  [unwired: 2 in, 2 out]
            n219 = invoke on="调用节点" class="CCamera" method="SetFloatValue"(reference=w35, error in=w34, "strKey"="ExposureTime", "fValue"=w26) -> (reference out=w29:refnum<k24>, error out=w28:errorcluster, "SetFloatValue"=w33:i32)  [unwired: 1 in, 2 out]
            n220 = Equal To 0?(x=w33) -> (x = 0?=w32:bool)
            n221 = case shown="假" w32 {
              frame False {
                n222 = One Button Dialog(message="Set ExposureTime Failed!") -> ()  [unwired: 1 in, 1 out]
              }
              frame True {
              }
            }
            n223 = property on="GrabbingStatus" class="Bool (严格)"() -> ("Value"=w31:bool)  [unwired: 2 in, 2 out]
            n224 = case shown="假" w31 {
              tunnel: w29 -> [w50 _]
              tunnel: w28 -> [w49 _]
              frame False {
                n225 = property on="PixelFormat" class="DigNum (严格)"() -> ("Value"=w51:u32)  [unwired: 2 in, 2 out]
                n226 = invoke on="调用节点" class="CCamera" method="SetEnumValue"(reference=w50, error in=w49, "strKey"="PixelFormat", "nValue"=w51) -> ("SetEnumValue"=w52:i32)  [unwired: 1 in, 4 out]
                n227 = Equal To 0?(x=w52) -> (x = 0?=w53:bool)
                n228 = case shown="假" w53 {
                  frame False {
                    n229 = One Button Dialog(message="Set PixelFormat Failed!") -> ()  [unwired: 1 in, 1 out]
                  }
                  frame True {
                  }
                }
              }
              frame True {
              }
            }
          }
        }
      }
    }
    n230 = case shown="假" "TriggerSoftWare" {
      frame False {
      }
      frame True {
        n231 = local read "CCamera"() -> (w196:refnum<k24>)
        n232 = invoke class="CCamera" method="IsDeviceConnected"(reference=w196) -> (reference out=w195:refnum<k24>, error out=w194:errorcluster, "IsDeviceConnected"=w193:bool)  [unwired: 2 in]
        n233 = case shown="真" w193 {
          tunnel: w195 -> [_ w199]
          tunnel: w194 -> [_ w198]
          frame False {
          }
          frame True {
            n234 = invoke class="CCamera" method="SetCommandValue"(reference=w199, error in=w198, "strKey"="TriggerSoftware") -> ("SetCommandValue"=w200:i32)  [unwired: 1 in, 3 out]
            n235 = Equal To 0?(x=w200) -> (x = 0?=w201:bool)
            n236 = case shown="假" w201 {
              frame False {
                n237 = One Button Dialog(message="Trigger Failed") -> ()  [unwired: 1 in, 1 out]
              }
              frame True {
                n238 = One Button Dialog(message="SoftWare Trigger Once Success!") -> ()  [unwired: 1 in, 1 out]
              }
            }
          }
        }
      }
    }
    n239 = case shown="真" "AcquisitionStop" {
      frame False {
      }
      frame True {
        n240 = local read "CCamera"() -> (w175:refnum<k24>)
        n241 = invoke class="CCamera" method="StopGrabbing"(reference=w175) -> (error out=w172:errorcluster, "StopGrabbing"=w173:i32)  [unwired: 2 in, 1 out]
        n242 = Equal To 0?(x=w173) -> (x = 0?=w174:bool)
        n243 = case shown="真" w174 {
          tunnel: w172 -> [_ w188]
          frame False {
            n244 = One Button Dialog(message="Stop Grabbing Filed!") -> ()  [unwired: 1 in, 1 out]
          }
          frame True {
            n245 = property on="GrabbingStatus" class="Bool (严格)"(error in=w188, "Value"=FALSE) -> (error out=w187:errorcluster)  [unwired: 1 in, 1 out]
            n246 = property on="AcquisitionStart" class="Bool"(error in=w187, "DisabledEnum"=T3."Enabled" ("禁用")) -> (error out=w191:errorcluster)  [unwired: 1 in, 1 out]
            n247 = property on="AcquisitionStop" class="Bool"(error in=w191, "DisabledEnum"=T3."Disabled and Grayed Out" ("禁用")) -> (error out=w192:errorcluster)  [unwired: 1 in, 1 out]
            n248 = property on="TriggerSoftWare" class="Bool"(error in=w192, "DisabledEnum"=T3."Disabled and Grayed Out" ("禁用")) -> (error out=w179:errorcluster)  [unwired: 1 in, 1 out]
            n249 = property on="PixelFormat" class="DigNum (严格)"(error in=w179, "DisabledEnum"=T3."Enabled" ("禁用")) -> (error out=w178:errorcluster)  [unwired: 1 in, 1 out]
            n250 = property on="Height" class="DigNum (严格)"(error in=w178, "DisabledEnum"=T3."Enabled" ("禁用")) -> (error out=w185:errorcluster)  [unwired: 1 in, 1 out]
            n251 = property on="PayloadSize" class="DigNum (严格)"(error in=w185, "DisabledEnum"=T3."Enabled" ("禁用")) -> (error out=w184:errorcluster)  [unwired: 1 in, 1 out]
            n252 = property on="Width" class="DigNum (严格)"(error in=w184, "DisabledEnum"=T3."Enabled" ("禁用")) -> ()  [unwired: 1 in, 2 out]
          }
        }
      }
    }
  }
  n253 = case shown="真" w7 {
    frame False {
    }
    frame True {
      w482 = T3."Disabled and Grayed Out" ("禁用")
      n254 = local read "CCamera"() -> (w487:refnum<k24>)
      n255 = invoke class="CCamera" method="IsDeviceConnected"(reference=w487) -> (reference out=w486:refnum<k24>, error out=w483:errorcluster, "IsDeviceConnected"=w485:bool)  [unwired: 2 in]
      n256 = property on="OpenSatatus" class="Bool (严格)"() -> ("Value"=w484:bool)  [unwired: 2 in, 2 out]
      n257 = Or(x=w485, y=w484) -> (x .or. y?=w488:bool)
      n258 = case shown="真" w488 {
        tunnel: w486 -> [_ w513]
        tunnel: w483 -> [_ w512]
        frame False {
        }
        frame True {
          n259 = invoke class="CCamera" method="CloseDevice"(reference=w513, error in=w512) -> (reference out=w515:refnum<k24>, error out=w514:errorcluster)  [unwired: 1 in, 1 out]
          n260 = invoke class="CCamera" method="DestroyHandle"(reference=w515, error in=w514) -> ()  [unwired: 1 in, 3 out]
        }
      }
      n261 = property on="OpenDevice" class="Bool"("DisabledEnum"=T3."Enabled" ("禁用")) -> (error out=w508:errorcluster)  [unwired: 2 in, 1 out]
      n262 = property on="CloseDevice" class="Bool"(error in=w508, "DisabledEnum"=T3."Disabled and Grayed Out" ("禁用")) -> (error out=w507:errorcluster)  [unwired: 1 in, 1 out]
      n263 = property on="TriggerSoftWare" class="Bool"(error in=w507, "DisabledEnum"=T3."Disabled and Grayed Out" ("禁用")) -> (error out=w506:errorcluster)  [unwired: 1 in, 1 out]
      n264 = property on="AcquisitionStart" class="Bool"(error in=w506, "DisabledEnum"=T3."Disabled and Grayed Out" ("禁用")) -> (error out=w505:errorcluster)  [unwired: 1 in, 1 out]
      n265 = property on="AcquisitionStop" class="Bool"(error in=w505, "DisabledEnum"=T3."Disabled and Grayed Out" ("禁用")) -> (error out=w504:errorcluster)  [unwired: 1 in, 1 out]
      n266 = property on="Continuous" class="Bool"(error in=w504, "DisabledEnum"=T3."Disabled and Grayed Out" ("禁用")) -> (error out=w503:errorcluster)  [unwired: 1 in, 1 out]
      n267 = property on="TriggerMode" class="Bool"(error in=w503, "DisabledEnum"=T3."Disabled and Grayed Out" ("禁用")) -> (error out=w502:errorcluster)  [unwired: 1 in, 1 out]
      n268 = property on="ExposureTime" class="DigNum (严格)"(error in=w502, "DisabledEnum"=T3."Disabled and Grayed Out" ("禁用")) -> (error out=w501:errorcluster)  [unwired: 1 in, 1 out]
      n269 = property on="Gain" class="DigNum (严格)"(error in=w501, "DisabledEnum"=T3."Disabled and Grayed Out" ("禁用")) -> (error out=w491:errorcluster)  [unwired: 1 in, 1 out]
      n270 = property on="PixelFormat" class="DigNum (严格)"(error in=w491, "DisabledEnum"=w482) -> (error out=w481:errorcluster)  [unwired: 1 in, 1 out]
      n271 = property on="GetParam" class="Bool"(error in=w481, "DisabledEnum"=w482) -> (error out=w480:errorcluster)  [unwired: 1 in, 1 out]
      n272 = property on="SetParam" class="Bool"(error in=w480, "DisabledEnum"=w482) -> (error out=w479:errorcluster)  [unwired: 1 in, 1 out]
      n273 = property on="OpenSatatus" class="Bool (严格)"(error in=w479, "Value"=FALSE) -> (error out=w511:errorcluster)  [unwired: 1 in, 1 out]
      n274 = property on="GrabbingStatus" class="Bool (严格)"(error in=w511, "Value"=FALSE) -> (error out=w490:errorcluster)  [unwired: 1 in, 1 out]
      n275 = property on="DeviceNum" class="DigNum (严格)"(error in=w490, "Value"=0) -> ()  [unwired: 1 in, 2 out]
    }
  }
